vi "Test Beep Actor.vi"() -> ()   [LabVIEW 2016, in "CS++BeepActor.lvlib"]
doc: "Test Beep Actor"
uses:
  CS++BeepActor.lvlib
  Beep.lvclass
  C:/User/Brand/LVP/TASCA/UTCS/Packages/CSPP_Core/Actors/CS++BaseActor/CS++BaseActor.lvclass
  C:/Program Files (x86)/National Instruments/LabVIEW 2016/vi.lib/ActorFramework/Actor/Actor.lvclass
  CSPP_Core/Actors/CS++BaseActor/CS++BaseActor.lvclass/CS++BaseActor.ctl
  <vilib>/ActorFramework/Message Enqueuer/Message Enqueuer.lvclass/Message Enqueuer.ctl
  <vilib>/ActorFramework/Message Enqueuer/Enqueue.vi
  Beep Messages/Beep Msg/Beep Msg.lvclass
  C:/Program Files (x86)/National Instruments/LabVIEW 2016/vi.lib/ActorFramework/Message/Message.lvclass
  <vilib>/ActorFramework/Stop Msg/Stop Msg.lvclass
  <vilib>/ActorFramework/Message Priority Queue/Priority Enqueue.vi
  CSPP_Core/Actors/CS++BaseActor/CS++BaseActor.lvclass
  <vilib>/ActorFramework/Actor/Actor.lvclass
panel:
  out "Loop":i32
  in  "Loop Interval":dbl[unit]
  in  "Stop Button":bool
  in  "Polling Iterations":u32
  in  "Polling Interval":dbl[unit]=1.0
  in  "Duration":dbl[unit]=0.1
  in  "Frequency (440)":dbl[unit]=440.0
  in  "Use System Alert?":bool
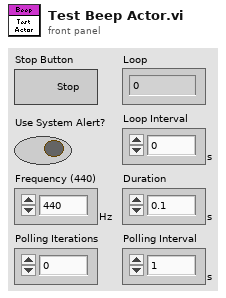
[diagram p1: front panel]
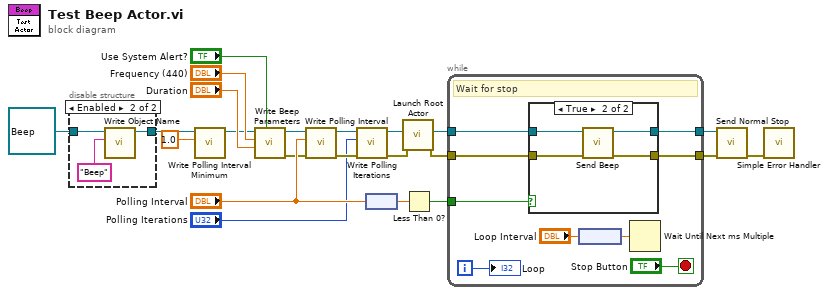
[diagram p0: block diagram]
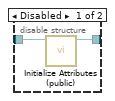
[diagram p2: hidden frame]
diagram:
  n1 = disable-structure shown="Enabled" {
    disable-tunnel: refnum<class "Beep.lvclass"> refnum ("CS++BeepActor.lvlib:Beep.lvclass") -> [w24 w27]
    disable-tunnel: [w23 w26] -> w3
    frame Disabled {
      n2 = call "Initialize Attributes (public).vi"("CS++BaseActor in"=w24) -> ("CS++BaseActor out"=w23:refnum<class "Beep.lvclass">)  [unwired: 8 in, 2 out]
    }
    frame Enabled {
      n3 = call "Write Object Name.vi"("Object Name"="Beep", "CS++BaseActor in"=w27) -> ("CS++BaseActor out"=w26:refnum<class "Beep.lvclass">)  [unwired: 8 in, 1 out]
    }
  }
  n4 = call "Write Polling Interval Minimum.vi"("Polling Interval Minimum"=dbl[unit] 1.0, "CS++BaseActor in"=w3) -> ("CS++BaseActor out"=w2:refnum<class "Beep.lvclass">)  [unwired: 8 in, 1 out]
  n5 = call "Write Beep Parameters.vi"("Use System Alert?"="Use System Alert?", "Duration"="Duration", "Frequency (440)"="Frequency (440)", "Beep in"=w2) -> ("error out"=w13:errorcluster, "Beep out"=w15:refnum<class "Beep.lvclass">)  [unwired: 6 in]
  n6 = call "Write Polling Interval.vi"("error in (no error)"=w13, "Polling Interval"="Polling Interval", "CS++BaseActor in"=w15) -> ("error out"=w11:errorcluster, "CS++BaseActor out"=w12:refnum<class "Beep.lvclass">)  [unwired: 7 in]
  n7 = call-dynamic "Write Polling Iterations.vi"("error in (no error)"=w11, "Polling Iterations"="Polling Iterations", "CS++BaseActor in"=w12) -> ("error out"=w8:errorcluster, "CS++BaseActor out"=w9:refnum<class "Beep.lvclass">)  [unwired: 7 in]
  n8 = node("Polling Interval") -> (w17:dbl)
  n9 = call <vilib>:"Launch Root Actor.vi"("error in (no error)"=w8, "Actor"=w9) -> ("error out"=w5:errorcluster, "Actor's Enqueuer"=w6:refnum<class "Message Enqueuer.lvclass">)  [unwired: 8 in]
  n10 = Less Than 0?(x=w17) -> (x < 0?=w16:bool)
  n11 = while {
    tunnel: [w32] -> w19
    tunnel: [w31] -> w18
    tunnel: w16 -> [w33]
    tunnel: w6 -> [w30]
    tunnel: w5 -> [w29]
    i -> [w28]
    stop <- "Stop Button" stop-if-true
    # "Wait for stop"
    n12 = case shown="True" w33 {
      tunnel: [w38 w42] -> w32
      tunnel: [w37 w41] -> w31
      tunnel: w30 -> [w38 w40]
      tunnel: w29 -> [w37 w39]
      frame False {
      }
      frame True {
        n13 = call "Send Beep.vi"("error in (no error)"=w39, "Message Enqueuer"=w40) -> ("error out"=w41:errorcluster, "Message Enqueuer out"=w42:refnum<class "Message Enqueuer.lvclass">)  [unwired: 8 in]
      }
    }
    n14 = node("Loop Interval") -> (w34:dbl)
    n15 = Wait Until Next ms Multiple(millisecond multiple=w34) -> ()  [unwired: 1 out]
    "Loop" <- w28
  }
  n16 = call <vilib>:"Send Normal Stop.vi"("error in (no error)"=w18, "Message Enqueuer"=w19) -> ("error out"=w7:errorcluster)  [unwired: 9 in]
  n17 = call <vilib>:"Simple Error Handler.vi"("error in (no error)"=w7) -> ()  [unwired: 4 in, 5 out]
